vi "Close.vi"(8 "error in (no error)":errorcluster, 11 "LT_UpgradeFlash in":refnum<class "LT_UpgradeFlash.lvclass">) -> (0 "error out":errorcluster, 3 "LT_UpgradeFlash out":refnum<class "LT_UpgradeFlash.lvclass">)   [LabVIEW 2017, in "LT_UpgradeFlash.lvclass"]
uses:
  LT_UpgradeFlash.lvclass
  D:/Project/Tymphany/LT_UpgradeFlash/New_Lib/LT_UpgradeFlash_dll/LT_UpgradeFlash_dll/bin/Debug/LT_UpgradeFlash_dll.dll
  New_Lib/LT_UpgradeFlash_dll/LT_UpgradeFlash_dll/bin/Debug/LT_UpgradeFlash_dll.dll
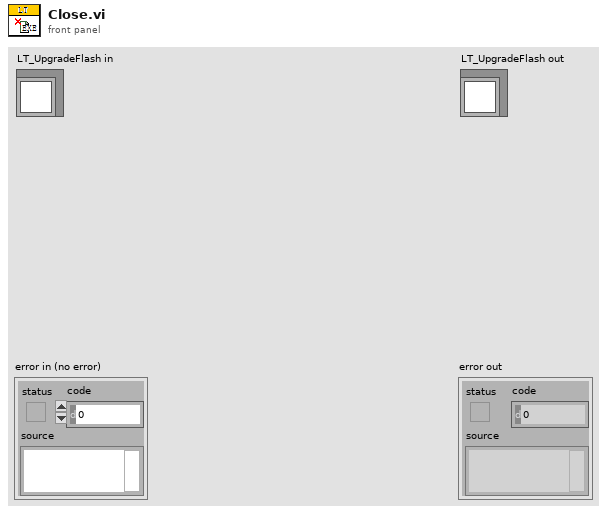
[diagram p1: front panel]
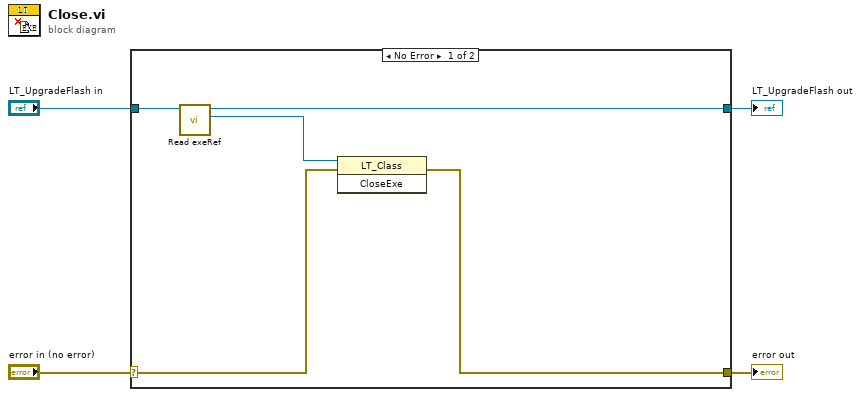
[diagram p0: block diagram]
diagram:
  n1 = case shown="No Error" "error in (no error)" {
    selector: "error in (no error)" -> [w6 w11]
    tunnel: [w5 w11] -> w3
    tunnel: [w8 w10] -> w1
    tunnel: "LT_UpgradeFlash in" -> [w9 w10]
    frame No Error {
      n2 = call-dynamic "Read exeRef.vi"("LT_UpgradeFlash in"=w9) -> ("exeRef"=w7:refnum<k24>, "LT_UpgradeFlash out"=w8:refnum<class "LT_UpgradeFlash.lvclass">)  [unwired: 8 in, 1 out]
      n3 = invoke class="LT_Class" method="CloseExe"(reference=w7, error in=w6) -> (error out=w5:errorcluster)  [unwired: 1 in, 2 out]
    }
    frame Error {
    }
  }
  "error out" <- w3
  "LT_UpgradeFlash out" <- w1
